vi "PurePursuitMain.vi"() -> ()   [LabVIEW 2016]
panel:
  in  "tolerance":dbl=0.001
  in  "B":dbl=0.95
  in  "A":dbl=0.05
  out "Vel Right":cluster{"r":dbl, "dx/dt":dbl}(graph)={"r"=83.40643380585193, "dx/dt"=58.28542836331929}
  in  "Kv":dbl=0.02
  in  "FFV":dbl=0.0082
  out "Vel Left":cluster{"l":dbl, "dx/dt":dbl}(graph)={"l"=86.59356619414807, "dx/dt"=58.34465005848233}
  in  "Vel":dbl=85.0
  out "Robot":T1={"Point"={"x"=4.605957313690988e-16, "y"=7.522099134048827}, "Angle"=0.0} {"Angle" scale=0.0..360.0}
  in  "LookAhead":dbl(slide)=29.212121212121215 scale=1.0..50.0
  in  "Path":cluster{"x":dbl, "y":dbl}[](array[cluster])=[{"x"=0.0, "y"=10.0}, {"x"=0.0, "y"=80.0}, {"x"=125.0, "y"=175.0}, {"x"=135.0, "y"=125.0}, {"x"=150.0, "y"=50.0}]
  out "Graph":cluster{cluster{"x":dbl, "y":dbl}[]}[](graph)=[{[{"x"=0.0, "y"=10.0}, {"x"=0.051701429312950624, "y"=13.965985448706023}, {"x"=0.10612294642514128, "y"=17.930177040126097}, {"x"=0.16612580880902378, "y"=21.890690583740415}, {"x"=0.23488386148018742, "y"=25.845451594729347}, {"x"=0.31599126375152675, "y"=29.792088060490833}, {"x"=0.41374824216620343, "y"=33.72776767550008}, {"x"=0.5332810061243543, "y"=37.64915193016147}, {"x"=0.680871942304378, "y"=41.552063134003845}, {"x"=0.8643022495509501, "y"=45.43138799873055}, {"x"=1.0932262388701397, "y"=49.280802406127826}, {"x"=1.3796816586868879, "y"=53.09237249288416}, {"x"=1.7387441369020282, "y"=56.856157420003235}, {"x"=2.1893209073945368, "y"=60.559726548437574}, {"x"=2.755132214826423, "y"=64.18749632093224}, {"x"=3.465954758420349, "y"=67.71988062560382}, {"x"=4.359194676210529, "y"=71.13226000090671}, {"x"=5.481865545124856, "y"=74.39369005370528}, {"x"=6.893055034088953, "y"=77.46531880762663}, {"x"=8.667042737244042, "y"=80.40353406577233}, {"x"=10.729576922546107, "y"=83.23561773410393}, {"x"=13.02159550045327, "y"=85.98323077024014}, {"x"=15.496117148885444, "y"=88.66358004564886}, {"x"=18.115766614529115, "y"=91.29035199826704}, {"x"=20.850809582842555, "y"=93.87442018935342}, {"x"=23.677586625805123, "y"=96.42440604670617}, {"x"=26.577264432863693, "y"=98.94713518343809}, {"x"=29.53484349881226, "y"=101.44799925204275}, {"x"=32.538370775059185, "y"=103.93123745748123}, {"x"=35.578312897229786, "y"=106.40015851415966}, {"x"=38.647054802678745, "y"=108.85731761060897}, {"x"=41.73849766263062, "y"=111.30465402349618}, {"x"=44.84773650226558, "y"=113.74359270941692}, {"x"=47.97080159495668, "y"=116.1751157028741}, {"x"=51.10444994316637, "y"=118.59981107387374}, {"x"=54.245996044477316, "y"=121.0179013233199}, {"x"=57.39316829228435, "y"=123.42927017690519}, {"x"=60.54400031948651, "y"=125.83341845102478}, {"x"=63.69669874261317, "y"=128.22953965479346}, {"x"=66.84960476387458, "y"=130.6163044427327}, {"x"=70.00102690779786, "y"=132.99198312055785}, {"x"=73.14922477490526, "y"=135.35424447963445}, {"x"=76.2922874118856, "y"=137.69999428241914}, {"x"=79.42801670104431, "y"=140.02530901025062}, {"x"=82.5538348352245, "y"=142.3252146482104}, {"x"=85.6666516276454, "y"=144.59336901757405}, {"x"=88.7626884947956, "y"=146.82174115418044}, {"x"=91.8372777813876, "y"=149.00022643394232}, {"x"=94.8846249885476, "y"=151.11611367322465}, {"x"=97.89750645439092, "y"=153.15338966201176}, {"x"=100.86688464994579, "y"=155.09188574165626}, {"x"=103.7814288968114, "y"=156.90622923596476}, {"x"=106.62692042111716, "y"=158.5645228927272}, {"x"=109.38550736356778, "y"=160.0266664890128}, {"x"=112.03476632051058, "y"=161.24223604236417}, {"x"=114.54652084533129, "y"=162.14782298062747}, {"x"=116.88535577093474, "y"=162.66369669459115}, {"x"=119.00675568206331, "y"=162.68961951312068}, {"x"=120.85475669260597, "y"=162.09956807053646}, {"x"=122.48458926960659, "y"=160.830547230216}, {"x"=123.94074448419457, "y"=159.02220978656834}, {"x"=125.25857530755984, "y"=156.78581855581777}, {"x"=126.46615542853507, "y"=154.21010462567048}, {"x"=127.58575219606956, "y"=151.36593796167912}, {"x"=128.63500179066165, "y"=148.31005976915256}, {"x"=129.627840380301, "y"=145.08807199750285}, {"x"=130.57523605950027, "y"=141.73683741524087}, {"x"=131.48576434747548, "y"=138.28641677371667}, {"x"=132.36606000600983, "y"=134.76164833894563}, {"x"=133.22116711196693, "y"=131.1834548956147}, {"x"=134.05480420005767, "y"=127.56994634084576}, {"x"=134.8695591873615, "y"=123.93737432442387}, {"x"=135.6774487051665, "y"=120.24887278641769}, {"x"=136.4797051171479, "y"=116.51674866916316}, {"x"=137.2772650467155, "y"=112.75101363793085}, {"x"=138.07081843920855, "y"=108.9599103562562}, {"x"=138.86084418801016, "y"=105.15034571605393}, {"x"=139.64763490471236, "y"=101.32825407095842}, {"x"=140.43131246853918, "y"=97.49890974619845}, {"x"=141.211834937656, "y"=93.66720519644947}, {"x"=141.98899472576807, "y"=89.83790914577169}, {"x"=142.76240768592592, "y"=86.01591793819303}, {"x"=143.53149260582566, "y"=82.20651313718191}, {"x"=144.29544030106356, "y"=78.41563901108485}, {"x"=145.05317089241086, "y"=74.65021478920546}, {"x"=145.80327705168938, "y"=70.91849842939382}, {"x"=146.543950118212, "y"=67.23052121338807}, {"x"=147.27288506004854, "y"=63.59861601537153}, {"x"=147.98715920868986, "y"=60.03806686900466}, {"x"=148.68307840027836, "y"=56.56791380172213}, {"x"=149.35598248299164, "y"=53.211955140299544}, {"x"=150.0, "y"=50.0}]}, {[{"x"=4.605957313690988e-16, "y"=7.522099134048827}, {"x"=1.0729191309427754e-15, "y"=17.522099134048826}]}, {[{"x"=0.5332810061243543, "y"=37.64915193016147}]}, {[{"x"=29.212121212121215, "y"=7.522099134048827}, {"x"=29.15447776378345, "y"=9.356343401511193}, {"x"=28.981774911125964, "y"=11.183348744836382}, {"x"=28.69469423340776, "y"=12.99590480861363}, {"x"=28.294368706909104, "y"=14.786858262137313}, {"x"=27.78237823359176, "y"=16.54914103033517}, {"x"=27.16074340594771, "y"=18.27579818823154}, {"x"=26.431917532643723, "y"=19.96001540885883}, {"x"=25.598776956432864, "y"=21.595145856292877}, {"x"=24.664609702543714, "y"=23.1747364176777}, {"x"=23.63310250234695, "y"=24.6925531707138}, {"x"=22.508326243510933, "y"=26.14260598610146}, {"x"=21.294719904067904, "y"=27.519172167844463}, {"x"=19.997073033795633, "y"=28.81681903811673}, {"x"=18.620506852052632, "y"=30.030425377559762}, {"x"=17.17045403666497, "y"=31.155201636395777}, {"x"=15.65263728362887, "y"=32.186708836592544}, {"x"=14.073046722244044, "y"=33.120876090481694}, {"x"=12.437916274810002, "y"=33.95401666669255}, {"x"=10.753699054182713, "y"=34.68284253999654}, {"x"=9.027041896286345, "y"=35.30447736764059}, {"x"=7.264759128088485, "y"=35.816467840957934}, {"x"=5.473805674564803, "y"=36.21679336745659}, {"x"=3.6612496107875554, "y"=36.50387404517479}, {"x"=1.834244267462365, "y"=36.67657689783228}, {"x"=-4.237071645262047e-15, "y"=36.73422034617004}, {"x"=-1.834244267462367, "y"=36.67657689783228}, {"x"=-3.6612496107875576, "y"=36.50387404517479}, {"x"=-5.47380567456481, "y"=36.21679336745658}, {"x"=-7.264759128088487, "y"=35.816467840957934}, {"x"=-9.027041896286347, "y"=35.30447736764059}, {"x"=-10.753699054182714, "y"=34.682842539996535}, {"x"=-12.437916274810004, "y"=33.95401666669255}, {"x"=-14.073046722244053, "y"=33.12087609048169}, {"x"=-15.652637283628879, "y"=32.18670883659254}, {"x"=-17.17045403666497, "y"=31.155201636395777}, {"x"=-18.620506852052635, "y"=30.030425377559762}, {"x"=-19.997073033795637, "y"=28.816819038116726}, {"x"=-21.294719904067907, "y"=27.519172167844456}, {"x"=-22.50832624351094, "y"=26.142605986101454}, {"x"=-23.633102502346947, "y"=24.692553170713804}, {"x"=-24.664609702543714, "y"=23.1747364176777}, {"x"=-25.598776956432864, "y"=21.595145856292874}, {"x"=-26.431917532643727, "y"=19.960015408858826}, {"x"=-27.160743405947713, "y"=18.275798188231537}, {"x"=-27.782378233591764, "y"=16.54914103033516}, {"x"=-28.294368706909104, "y"=14.786858262137315}, {"x"=-28.69469423340776, "y"=12.99590480861363}, {"x"=-28.981774911125964, "y"=11.183348744836376}, {"x"=-29.15447776378345, "y"=9.356343401511186}, {"x"=-29.212121212121215, "y"=7.522099134048817}, {"x"=-29.15447776378345, "y"=5.687854866586461}, {"x"=-28.981774911125964, "y"=3.860849523261271}, {"x"=-28.694694233407755, "y"=2.048293459484018}, {"x"=-28.294368706909104, "y"=0.2573400059603346}, {"x"=-27.78237823359176, "y"=-1.5049427622375253}, {"x"=-27.160743405947706, "y"=-3.231599920133898}, {"x"=-26.431917532643723, "y"=-4.915817140761175}, {"x"=-25.59877695643286, "y"=-6.550947588195224}, {"x"=-24.66460970254371, "y"=-8.130538149580051}, {"x"=-23.633102502346944, "y"=-9.648354902616155}, {"x"=-22.50832624351093, "y"=-11.098407718003816}, {"x"=-21.294719904067904, "y"=-12.47497389974681}, {"x"=-19.997073033795633, "y"=-13.772620770019078}, {"x"=-18.62050685205263, "y"=-14.986227109462114}, {"x"=-17.170454036664978, "y"=-16.11100336829812}, {"x"=-15.652637283628863, "y"=-17.142510568494895}, {"x"=-14.073046722244047, "y"=-18.07667782238404}, {"x"=-12.437916274809988, "y"=-18.909818398594908}, {"x"=-10.75369905418271, "y"=-19.638644271898887}, {"x"=-9.027041896286347, "y"=-20.260279099542934}, {"x"=-7.264759128088475, "y"=-20.77226957286028}, {"x"=-5.473805674564804, "y"=-21.172595099358933}, {"x"=-3.661249610787539, "y"=-21.459675777077138}, {"x"=-1.8342442674623614, "y"=-21.632378629734625}, {"x"=-4.905583879440213e-15, "y"=-21.69002207807239}, {"x"=1.8342442674623771, "y"=-21.632378629734625}, {"x"=3.6612496107875545, "y"=-21.459675777077138}, {"x"=5.4738056745648205, "y"=-21.17259509935893}, {"x"=7.264759128088491, "y"=-20.772269572860278}, {"x"=9.027041896286338, "y"=-20.260279099542938}, {"x"=10.753699054182723, "y"=-19.63864427189888}, {"x"=12.43791627481, "y"=-18.9098183985949}, {"x"=14.07304672224406, "y"=-18.076677822384035}, {"x"=15.652637283628877, "y"=-17.142510568494885}, {"x"=17.170454036664992, "y"=-16.111003368298114}, {"x"=18.620506852052642, "y"=-14.986227109462103}, {"x"=19.997073033795633, "y"=-13.772620770019078}, {"x"=21.29471990406791, "y"=-12.474973899746796}, {"x"=22.50832624351094, "y"=-11.098407718003806}, {"x"=23.63310250234696, "y"=-9.64835490261613}, {"x"=24.66460970254372, "y"=-8.130538149580037}, {"x"=25.598776956432864, "y"=-6.550947588195222}, {"x"=26.43191753264373, "y"=-4.915817140761162}, {"x"=27.160743405947713, "y"=-3.2315999201338856}, {"x"=27.782378233591768, "y"=-1.5049427622374987}, {"x"=28.294368706909108, "y"=0.25734000596034967}, {"x"=28.69469423340776, "y"=2.0482934594840208}, {"x"=28.981774911125964, "y"=3.860849523261286}, {"x"=29.15447776378345, "y"=5.687854866586464}, {"x"=29.212121212121215, "y"=7.522099134048846}]}, {[{"x"=1600.1845479429587, "y"=7.522099134048827}, {"x"=1598.6057486039713, "y"=57.76030868810775}, {"x"=1593.875581386715, "y"=107.80025098071157}, {"x"=1586.0127141001885, "y"=157.44444122070638}, {"x"=1575.0481778893695, "y"=206.4969564694881}, {"x"=1561.025244769462, "y"=254.76420885933234}, {"x"=1543.9992568510215, "y"=302.05570959626647}, {"x"=1524.037407929928, "y"=348.18482073231337}, {"x"=1501.2184783041716, "y"=392.96949174020517}, {"x"=1475.6325238640084, "y"=436.2329779836439}, {"x"=1447.3805206825027, "y"=477.80453824763333}, {"x"=1416.5739665090991, "y"=517.5201085760509}, {"x"=1383.3344407389445, "y"=555.2229497571286}, {"x"=1347.793124594559, "y"=590.7642659015141}, {"x"=1310.0902834134813, "y"=624.0037916716686}, {"x"=1270.3747130850638, "y"=654.8103458450721}, {"x"=1228.8031528210745, "y"=683.0623490265779}, {"x"=1185.5396665776357, "y"=708.6483034667414}, {"x"=1140.7549955697439, "y"=731.4672330924975}, {"x"=1094.625884433697, "y"=751.429082013591}, {"x"=1047.3343836967629, "y"=768.4550699320315}, {"x"=999.0671313069186, "y"=782.4780030519391}, {"x"=950.0146160581369, "y"=793.4425392627581}, {"x"=900.370425818142, "y"=801.3054065492845}, {"x"=850.3304835255382, "y"=806.0355737665408}, {"x"=800.0922739714792, "y"=807.6143731055282}, {"x"=749.8540644174204, "y"=806.0355737665408}, {"x"=699.8141221248165, "y"=801.3054065492844}, {"x"=650.1699318848216, "y"=793.442539262758}, {"x"=601.11741663604, "y"=782.4780030519391}, {"x"=552.8501642461957, "y"=768.4550699320315}, {"x"=505.5586635092617, "y"=751.4290820135909}, {"x"=459.4295523732148, "y"=731.4672330924974}, {"x"=414.6448813653229, "y"=708.6483034667411}, {"x"=371.3813951218841, "y"=683.0623490265779}, {"x"=329.80983485789494, "y"=654.8103458450721}, {"x"=290.09426452947724, "y"=624.0037916716686}, {"x"=252.3914233483996, "y"=590.764265901514}, {"x"=216.85010720401397, "y"=555.2229497571284}, {"x"=183.61058143385947, "y"=517.5201085760508}, {"x"=152.80402726045622, "y"=477.80453824763345}, {"x"=124.55202407895035, "y"=436.2329779836439}, {"x"=98.96606963878696, "y"=392.9694917402051}, {"x"=76.14714001303071, "y"=348.1848207323132}, {"x"=56.18529109193719, "y"=302.0557095962663}, {"x"=39.159303173496596, "y"=254.76420885933211}, {"x"=25.136370053589076, "y"=206.49695646948814}, {"x"=14.17183384277007, "y"=157.44444122070632}, {"x"=6.308966556243718, "y"=107.80025098071143}, {"x"=1.5787993389874373, "y"=57.760308688107564}, {"x"=0.0, "y"=7.5220991340485694}, {"x"=1.5787993389874373, "y"=-42.71611042001007}, {"x"=6.308966556243718, "y"=-92.75605271261392}, {"x"=14.171833842770184, "y"=-142.40024295260883}, {"x"=25.136370053589076, "y"=-191.45275820139065}, {"x"=39.15930317349671, "y"=-239.72001059123494}, {"x"=56.1852910919373, "y"=-287.01151132816915}, {"x"=76.14714001303082, "y"=-333.1406224642157}, {"x"=98.96606963878708, "y"=-377.9252934721076}, {"x"=124.55202407895035, "y"=-421.1887797155464}, {"x"=152.80402726045634, "y"=-462.7603399795359}, {"x"=183.6105814338598, "y"=-502.4759103079535}, {"x"=216.85010720401408, "y"=-540.1787514890309}, {"x"=252.3914233483997, "y"=-575.7200676334164}, {"x"=290.0942645294774, "y"=-608.959593403571}, {"x"=329.8098348578947, "y"=-639.7661475769743}, {"x"=371.3813951218845, "y"=-668.0181507584804}, {"x"=414.644881365323, "y"=-693.6041051986435}, {"x"=459.42955237321524, "y"=-716.4230348244}, {"x"=505.55866350926186, "y"=-736.3848837454933}, {"x"=552.8501642461957, "y"=-753.4108716639338}, {"x"=601.1174166360404, "y"=-767.4338047838414}, {"x"=650.1699318848218, "y"=-778.3983409946604}, {"x"=699.814122124817, "y"=-786.2612082811868}, {"x"=749.8540644174205, "y"=-790.9913754984431}, {"x"=800.0922739714792, "y"=-792.5701748374305}, {"x"=850.3304835255385, "y"=-790.9913754984431}, {"x"=900.370425818142, "y"=-786.2612082811868}, {"x"=950.0146160581373, "y"=-778.3983409946603}, {"x"=999.0671313069188, "y"=-767.4338047838414}, {"x"=1047.3343836967626, "y"=-753.4108716639339}, {"x"=1094.6258844336971, "y"=-736.3848837454932}, {"x"=1140.7549955697439, "y"=-716.4230348243998}, {"x"=1185.5396665776361, "y"=-693.6041051986434}, {"x"=1228.8031528210745, "y"=-668.0181507584801}, {"x"=1270.3747130850643, "y"=-639.766147576974}, {"x"=1310.0902834134818, "y"=-608.9595934035707}, {"x"=1347.793124594559, "y"=-575.7200676334164}, {"x"=1383.334440738945, "y"=-540.1787514890306}, {"x"=1416.5739665090991, "y"=-502.47591030795326}, {"x"=1447.3805206825027, "y"=-462.7603399795353}, {"x"=1475.6325238640086, "y"=-421.18877971554605}, {"x"=1501.2184783041716, "y"=-377.92529347210757}, {"x"=1524.0374079299281, "y"=-333.14062246421537}, {"x"=1543.9992568510215, "y"=-287.01151132816875}, {"x"=1561.0252447694622, "y"=-239.7200105912342}, {"x"=1575.0481778893695, "y"=-191.45275820139022}, {"x"=1586.0127141001885, "y"=-142.40024295260878}, {"x"=1593.875581386715, "y"=-92.75605271261352}, {"x"=1598.6057486039713, "y"=-42.716110420010004}, {"x"=1600.1845479429587, "y"=7.522099134049341}]}, {[{"x"=0.0, "y"=10.0}, {"x"=2.4492935982947064e-16, "y"=14.0}, {"x"=4.898587196589413e-16, "y"=18.0}, {"x"=7.347880794884119e-16, "y"=22.0}, {"x"=9.797174393178826e-16, "y"=26.0}, {"x"=1.2246467991473533e-15, "y"=30.0}, {"x"=1.4695761589768238e-15, "y"=34.0}, {"x"=1.7145055188062944e-15, "y"=38.0}, {"x"=1.959434878635765e-15, "y"=42.0}, {"x"=2.204364238465236e-15, "y"=46.0}, {"x"=2.4492935982947065e-15, "y"=50.0}, {"x"=2.6942229581241772e-15, "y"=54.0}, {"x"=2.9391523179536475e-15, "y"=58.0}, {"x"=3.184081677783118e-15, "y"=62.0}, {"x"=3.429011037612589e-15, "y"=66.0}, {"x"=3.67394039744206e-15, "y"=70.0}, {"x"=3.91886975727153e-15, "y"=74.0}, {"x"=4.1637991171010006e-15, "y"=78.0}, {"x"=0.0, "y"=80.0}, {"x"=3.18464877649241, "y"=82.42033307013423}, {"x"=6.36929755298482, "y"=84.84066614026847}, {"x"=9.553946329477231, "y"=87.2609992104027}, {"x"=12.73859510596964, "y"=89.68133228053692}, {"x"=15.92324388246205, "y"=92.10166535067115}, {"x"=19.107892658954462, "y"=94.52199842080539}, {"x"=22.29254143544687, "y"=96.94233149093962}, {"x"=25.47719021193928, "y"=99.36266456107386}, {"x"=28.66183898843169, "y"=101.78299763120808}, {"x"=31.8464877649241, "y"=104.20333070134231}, {"x"=35.03113654141651, "y"=106.62366377147654}, {"x"=38.215785317908924, "y"=109.04399684161078}, {"x"=41.400434094401334, "y"=111.46432991174501}, {"x"=44.58508287089374, "y"=113.88466298187925}, {"x"=47.76973164738615, "y"=116.30499605201348}, {"x"=50.95438042387856, "y"=118.72532912214771}, {"x"=54.13902920037097, "y"=121.14566219228195}, {"x"=57.32367797686338, "y"=123.56599526241617}, {"x"=60.50832675335579, "y"=125.9863283325504}, {"x"=63.6929755298482, "y"=128.40666140268462}, {"x"=66.8776243063406, "y"=130.82699447281885}, {"x"=70.06227308283302, "y"=133.2473275429531}, {"x"=73.24692185932543, "y"=135.66766061308732}, {"x"=76.43157063581785, "y"=138.08799368322155}, {"x"=79.61621941231026, "y"=140.5083267533558}, {"x"=82.80086818880267, "y"=142.92865982349002}, {"x"=85.98551696529508, "y"=145.34899289362426}, {"x"=89.17016574178749, "y"=147.7693259637585}, {"x"=92.3548145182799, "y"=150.18965903389272}, {"x"=95.5394632947723, "y"=152.60999210402696}, {"x"=98.72411207126471, "y"=155.0303251741612}, {"x"=101.90876084775712, "y"=157.45065824429543}, {"x"=105.09340962424953, "y"=159.87099131442966}, {"x"=108.27805840074194, "y"=162.2913243845639}, {"x"=111.46270717723435, "y"=164.71165745469813}, {"x"=114.64735595372676, "y"=167.13199052483233}, {"x"=117.83200473021917, "y"=169.55232359496657}, {"x"=121.01665350671158, "y"=171.9726566651008}, {"x"=124.20130228320399, "y"=174.39298973523503}, {"x"=125.0, "y"=175.0}, {"x"=125.78446454055273, "y"=171.0776772972363}, {"x"=126.56892908110547, "y"=167.15535459447264}, {"x"=127.35339362165821, "y"=163.23303189170895}, {"x"=128.13785816221093, "y"=159.31070918894528}, {"x"=128.92232270276367, "y"=155.3883864861816}, {"x"=129.70678724331643, "y"=151.46606378341792}, {"x"=130.49125178386916, "y"=147.54374108065423}, {"x"=131.2757163244219, "y"=143.62141837789056}, {"x"=132.06018086497463, "y"=139.69909567512687}, {"x"=132.84464540552736, "y"=135.7767729723632}, {"x"=133.6291099460801, "y"=131.8544502695995}, {"x"=134.41357448663283, "y"=127.93212756683583}, {"x"=135.0, "y"=125.0}, {"x"=135.78446454055273, "y"=121.07767729723632}, {"x"=136.56892908110547, "y"=117.15535459447264}, {"x"=137.3533936216582, "y"=113.23303189170896}, {"x"=138.13785816221093, "y"=109.31070918894528}, {"x"=138.92232270276367, "y"=105.3883864861816}, {"x"=139.70678724331643, "y"=101.46606378341792}, {"x"=140.49125178386916, "y"=97.54374108065423}, {"x"=141.2757163244219, "y"=93.62141837789056}, {"x"=142.06018086497463, "y"=89.69909567512687}, {"x"=142.84464540552736, "y"=85.7767729723632}, {"x"=143.6291099460801, "y"=81.85445026959951}, {"x"=144.41357448663283, "y"=77.93212756683583}, {"x"=145.19803902718556, "y"=74.00980486407215}, {"x"=145.9825035677383, "y"=70.08748216130847}, {"x"=146.76696810829105, "y"=66.16515945854479}, {"x"=147.5514326488438, "y"=62.24283675578111}, {"x"=148.33589718939652, "y"=58.32051405301743}, {"x"=149.12036172994925, "y"=54.398191350253754}, {"x"=149.90482627050199, "y"=50.475868647490074}, {"x"=150.0, "y"=50.0}]}]
  # ".0082"
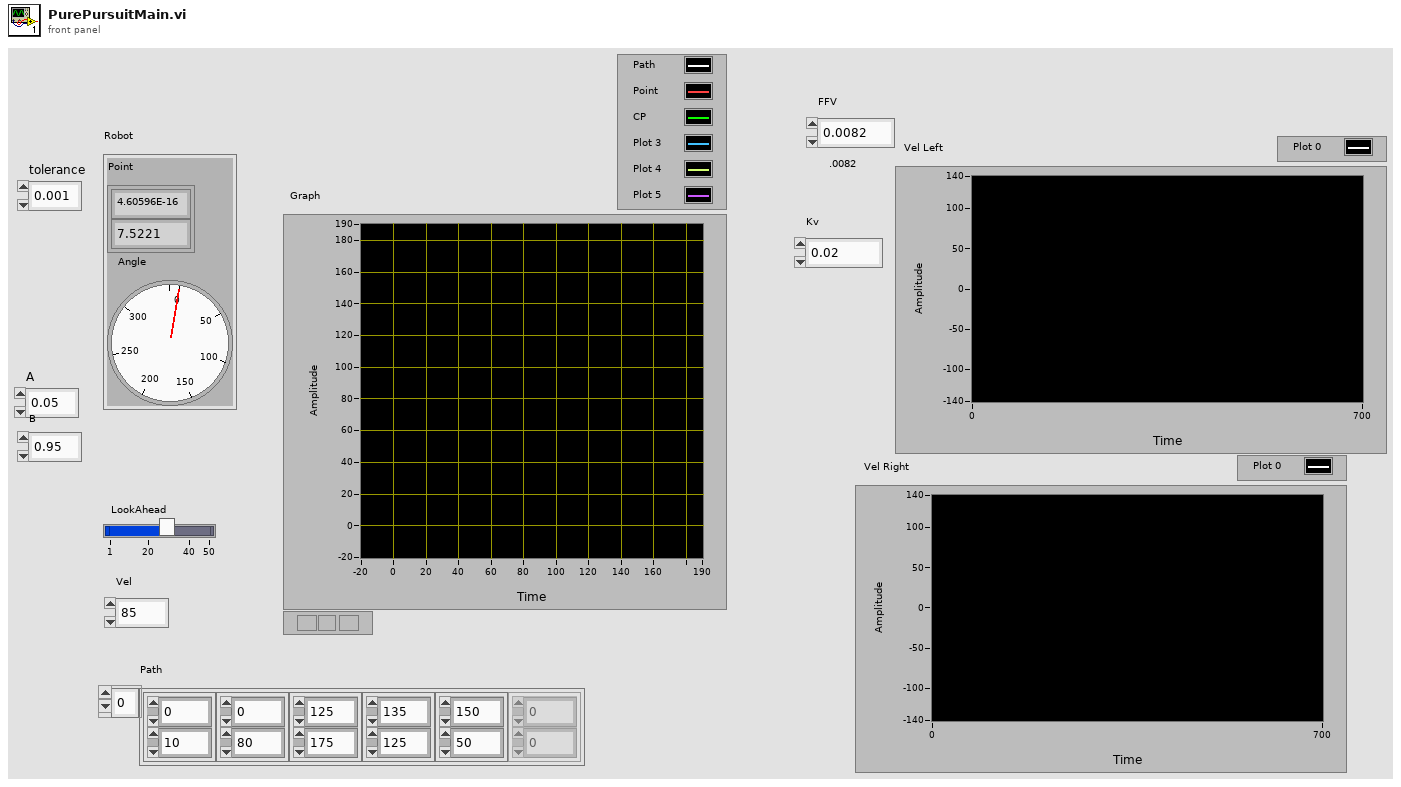
[diagram p1: front panel]
types:
  T1 = cluster{"Point":cluster{"x":dbl, "y":dbl}, "Angle":dbl}
  T2 = cluster{"Path out":cluster{"x":dbl, "y":dbl}[]}[]
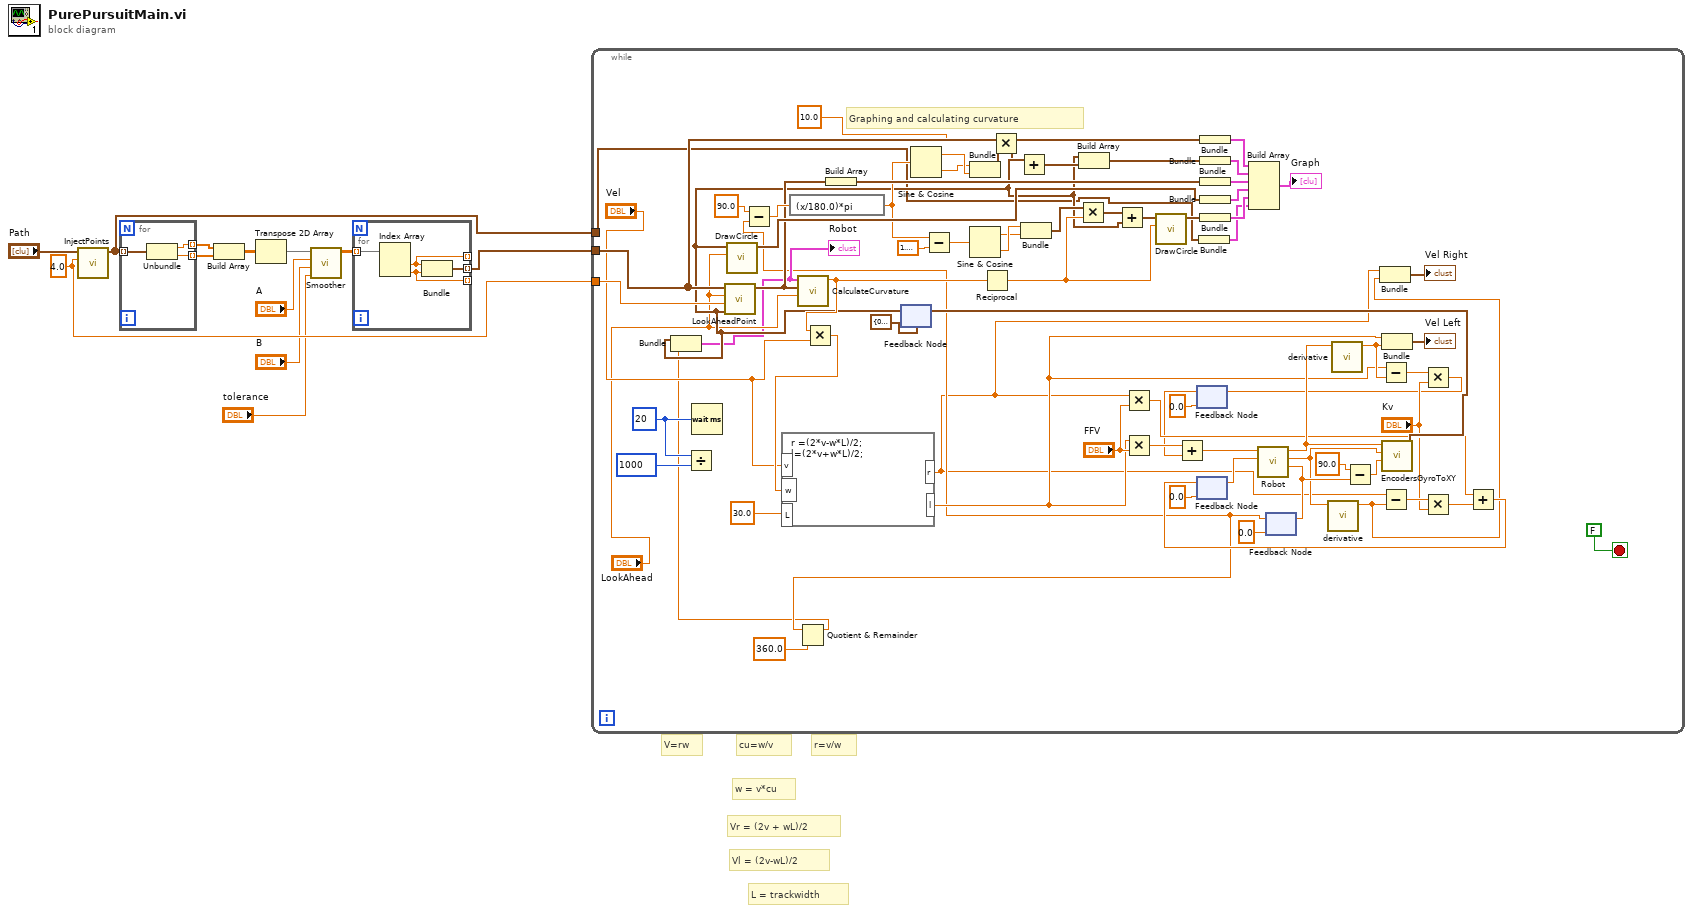
[diagram p0: block diagram]
diagram:
  w11 = 4.0 ("Distance")
  # "L = trackwidth"
  # "Vl = (2v-wL)/2"
  # "Vr = (2v + wL)/2"
  # "w = v*cu"
  # "cu=w/v"
  # "r=v/w"
  # "V=rw"
  n1 = call "InjectPoints.vi"("Distance"=w11, "Path"="Path") -> ("Path out"=w2:cluster{dbl, dbl}[])  [unwired: 9 in]
  n2 = for {
    tunnel: w2 -> [w15] mode=indexing
    tunnel: [w14] -> w10 mode=indexing
    tunnel: [w13] -> w9 mode=indexing
    n3 = Unbundle(w15) -> (w14:dbl, w13:dbl)
  }
  n4 = Build Array(w10, w9) -> (w8:dbl[][])
  n5 = Transpose 2D Array(2D array=w8) -> (transposed array=w7:dbl[][])
  n6 = call "Smoother.vi"("tolerance"="tolerance", "B"="B", "A"="A", "Array In"=w7) -> ("Smooth Array"=w6:dbl[][])  [unwired: 7 in]
  n7 = for {
    tunnel: w6 -> [w19] mode=indexing
    tunnel: [w18] -> _ mode=indexing
    tunnel: [w17] -> _ mode=indexing
    tunnel: [w16] -> w1 mode=indexing
    n8 = Index Array(array=w19) -> (element #1=w18:dbl, element #2=w17:dbl)  [unwired: 2 in]
    n9 = Bundle(w18, w17) -> (w16:cluster{dbl, dbl})  [unwired: 1 in]
  }
  n10 = while {
    tunnel: w1 -> [w88]
    tunnel: w11 -> [w79]
    tunnel: w2 -> [w20]
    stop <- FALSE stop-if-true
    w66 = u32 20 ("milliseconds to wait")
    # "Graphing and calculating curvature"
    n11 = Divide(x=w66, y=u32 1000) -> ()  [unwired: 1 out]
    n12 = Wait (ms)(milliseconds to wait=w66) -> ()  [unwired: 1 out]
    n13 = feedback #1(cluster{dbl, dbl} {0.0, 0.0} ("Location")) -> (w56:cluster{dbl, dbl})
    n14 = call "LookAheadPoint.vi"("Robot"=w56, "Spacing"=w79, "LookAhead"="LookAhead", "Path"=w88) -> ("Point"=w78:cluster{"x":dbl, "y":dbl})  [unwired: 7 in]
    n15 = call "DrawCircle.vi"("r"="LookAhead", "Center"=w56) -> ("Circle Graph"=w80:cluster{dbl, dbl}[])  [unwired: 9 in]
    n16 = Build Array(w78) -> (w90:cluster{"x":dbl, "y":dbl}[])
    n17 = feedback #2(0.0) -> (w37:dbl)
    n18 = feedback #3(0.0) -> (w33:dbl)
    n19 = Bundle("Path out"=w20) -> (w21:cluster{"Path out":cluster{dbl, dbl}[]})  [unwired: 1 in]
    n20 = Bundle(w88) -> (w91:cluster{cluster{dbl, dbl}[]})  [unwired: 1 in]
    n21 = Bundle(w90) -> (w89:cluster{cluster{"x":dbl, "y":dbl}[]})  [unwired: 1 in]
    n22 = Bundle("Circle Graph"=w80) -> (w81:cluster{"Circle Graph":cluster{dbl, dbl}[]})  [unwired: 1 in]
    n23 = feedback #4(0.0 ("Angle")) -> (w27:dbl)
    n24 = Subtract(x=90.0, y=w27) -> (x-y=w82:dbl)
    n25 = expression code="(x/180.0)*pi" ("degrees to radians")(w82) -> (w70:dbl)
    n26 = Quotient & Remainder(x=w27, y=360.0) -> (x-y*floor(x/y)=w26:dbl)  [unwired: 1 out]
    n27 = Bundle("Location"=w56, w26) -> (w29:cluster{"Location":cluster{dbl, dbl}, dbl})  [unwired: 1 in]
    "Robot" <- w29
    n28 = call "CalculateCurvature.vi"("Lookahead"="LookAhead", "Point"=w78, "Robot"=w29) -> ("Curvature"=w61:dbl)  [unwired: 8 in]
    n29 = Multiply(x=w61, y="Vel") -> (x*y=w59:dbl)
    n30 = formula code="r =(2*v-w*L)/2;\nl=(2*v+w*L)/2;"("L"=30.0 ("WheelBase"), "w"=w59, "v"="Vel") -> ("r"=w24:dbl, "l"=w43:dbl)
    n31 = Sine & Cosine(0:w70) -> (1:w87:dbl, 2:w86:dbl)
    n32 = Subtract(x=w70, y=1.5707963267948966) -> (x-y=w68:dbl)
    n33 = Bundle(w86, w87) -> (w48:cluster{dbl, dbl})  [unwired: 1 in]
    n34 = Sine & Cosine(0:w68) -> (1:w74:dbl, 2:w75:dbl)
    n35 = Reciprocal(x=w61) -> (1/x=w76:dbl)
    n36 = Multiply(x=10.0 ("Angle"), y=w48) -> (x*y=w47:cluster{dbl, dbl})
    n37 = Add(x=w56, y=w47) -> (x+y=w84:cluster{dbl, dbl})
    n38 = Bundle(w75, w74) -> (w73:cluster{dbl, dbl})  [unwired: 1 in]
    n39 = Multiply(x=w73, y=w76) -> (x*y=w72:cluster{dbl, dbl})
    n40 = Build Array(w56, w84) -> (w85:cluster{dbl, dbl}[])
    n41 = Add(x=w72, y=w56) -> (x+y=w71:cluster{dbl, dbl})
    n42 = Multiply(x=w24, y="FFV") -> (x*y=w52:dbl)
    n43 = Multiply(x=w43, y="FFV") -> (x*y=w39:dbl)
    n44 = call "DrawCircle.vi"("r"=w76, "Center"=w71) -> ("Circle Graph"=w22:cluster{dbl, dbl}[])  [unwired: 9 in]
    n45 = Add(x=w39, y=w37) -> (x+y=w62:dbl)
    n46 = Bundle(w85) -> (w92:cluster{cluster{dbl, dbl}[]})  [unwired: 1 in]
    n47 = Bundle("Circle Graph"=w22) -> (w77:cluster{"Circle Graph":cluster{dbl, dbl}[]})  [unwired: 1 in]
    n48 = Build Array(w91, w92, w89, w81, w77, w21) -> (→"Graph":T2)
    n49 = call "Robot.vi"("Right Value"=w33, "Left Value"=w62) -> ("Angle"=w50:dbl, "Right Distance"=w45:dbl, "Left Distance"=w58:dbl)  [unwired: 7 in]
    n50 = feedback-in #4(w50) -> ()
    n51 = call "derivative.vi"("x"=w45) -> ("dx/dt"=w23:dbl)  [unwired: 10 in]
    n52 = call "derivative.vi"("x"=w58) -> ("dx/dt"=w44:dbl)  [unwired: 10 in]
    n53 = Subtract(x=90.0, y=w50) -> (x-y=w49:dbl)
    n54 = Bundle("r"=w24, "dx/dt"=w23) -> (→"Vel Right":cluster{"r":dbl, "dx/dt":dbl})  [unwired: 1 in]
    n55 = Subtract(x=w43, y=w44) -> (x-y=w42:dbl)
    n56 = Subtract(x=w24, y=w23) -> (x-y=w41:dbl)
    n57 = Bundle("l"=w43, "dx/dt"=w44) -> (→"Vel Left":cluster{"l":dbl, "dx/dt":dbl})  [unwired: 1 in]
    n58 = call "EncodersGyroToXY.vi"("Angle (degrees)"=w49, "Right Distance"=w45, "Left Distance"=w58) -> ("Location"=w57:cluster{dbl, dbl})  [unwired: 7 in, 1 out]
    n59 = feedback-in #1(w57) -> ()
    n60 = Multiply(x=w42, y="Kv") -> (x*y=w38:dbl)
    n61 = feedback-in #2(w38) -> ()
    n62 = Multiply(x=w41, y="Kv") -> (x*y=w35:dbl)
    n63 = Add(x=w52, y=w35) -> (x+y=w34:dbl)
    n64 = feedback-in #3(w34) -> ()
  }
